vi "conv from ns to time clust.vi"(7 "time (nsec)":i64=1209600000) -> (8 "time cluster":T1={"day"=0, "hour"=0, "min"=0, "sec"=0, "msec"=1, "usec"=0, "nsec"=0}, 14 "nsec error":dbl)   [LabVIEW 2014]
doc: "This subvi converts a time in nsec to a typedefined cluster of: [days, hours (24), min, sec, msec, usec, and nsec]\n\nIt uses a I64 format for the time in nsec and thus is limited to 2^63-1 msec before rolling over.\n\nPaul K Dixon\nP350\nCSUSB Physics"
uses:
  typedefs/time cluster typedef.ctl
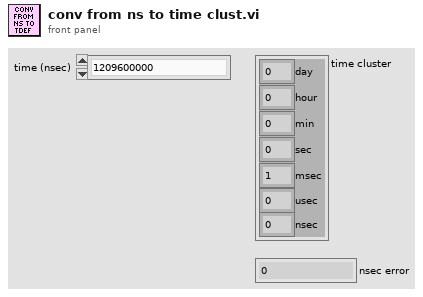
[diagram p1: front panel]
types:
  T1 = typedef "time cluster typedef.ctl" = cluster{"day":u32, "hour":u32, "min":u32, "sec":u32, "msec":u32, "usec":u32, "nsec":u32}
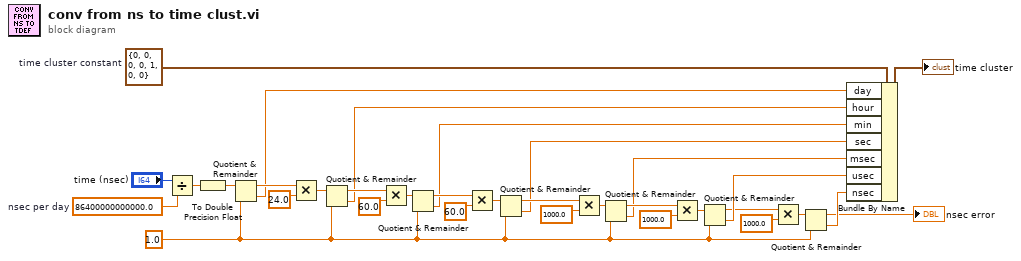
[diagram p0: block diagram]
diagram:
  w14 = T1 {"day"=0, "hour"=0, "min"=0, "sec"=0, "msec"=1, "usec"=0, "nsec"=0}  # time cluster constant
  w2 = 1.0 ("y")
  w32 = 86400000000000.0  # nsec per day
  n1 = Divide(x="time (nsec)", y=w32) -> (x/y=w31:dbl)
  n2 = To Double Precision Float(number=w31) -> (double precision float=w15:dbl)
  n3 = Quotient & Remainder(x=w15, y=w2) -> (x-y*floor(x/y)=w30:dbl, floor(x/y)=w12:dbl)
  n4 = Multiply(x=w30, y=24.0) -> (x*y=w28:dbl)
  n5 = Quotient & Remainder(x=w28, y=w2) -> (x-y*floor(x/y)=w27:dbl, floor(x/y)=w11:dbl)
  n6 = Multiply(x=w27, y=60.0) -> (x*y=w25:dbl)
  n7 = Quotient & Remainder(x=w25, y=w2) -> (x-y*floor(x/y)=w23:dbl, floor(x/y)=w10:dbl)
  n8 = Multiply(x=w23, y=60.0) -> (x*y=w22:dbl)
  n9 = Quotient & Remainder(x=w22, y=w2) -> (x-y*floor(x/y)=w19:dbl, floor(x/y)=w9:dbl)
  n10 = Multiply(x=w19, y=1000.0) -> (x*y=w21:dbl)
  n11 = Quotient & Remainder(x=w21, y=w2) -> (x-y*floor(x/y)=w17:dbl, floor(x/y)=w8:dbl)
  n12 = Multiply(x=w17, y=sgl 1000.0) -> (x*y=w16:dbl)
  n13 = Quotient & Remainder(x=w16, y=w2) -> (x-y*floor(x/y)=w5:dbl, floor(x/y)=w7:dbl)
  n14 = Multiply(x=w5, y=1000.0) -> (x*y=w4:dbl)
  n15 = Quotient & Remainder(x=w4, y=w2) -> (x-y*floor(x/y)=→"nsec error":dbl, floor(x/y)=w3:dbl)
  n16 = Bundle By Name(cluster=w14, "day"=w12, "hour"=w11, "min"=w10, "sec"=w9, "msec"=w8, "usec"=w7, "nsec"=w3) -> (→"time cluster":T1)
